vi "CPU_MEM_initialize_MEMs.vi"(8 "error in (no error)":errorcluster) -> (0 "error out":errorcluster)   [LabVIEW 2018]
uses:
  CPU_MEM_references.vi
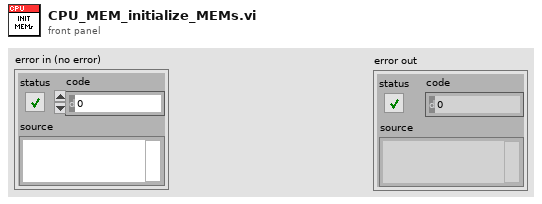
[diagram p1: front panel]
types:
  T1 = enum16{"init", "read DDR", "read PDR", "write DDR", "write PDR"}
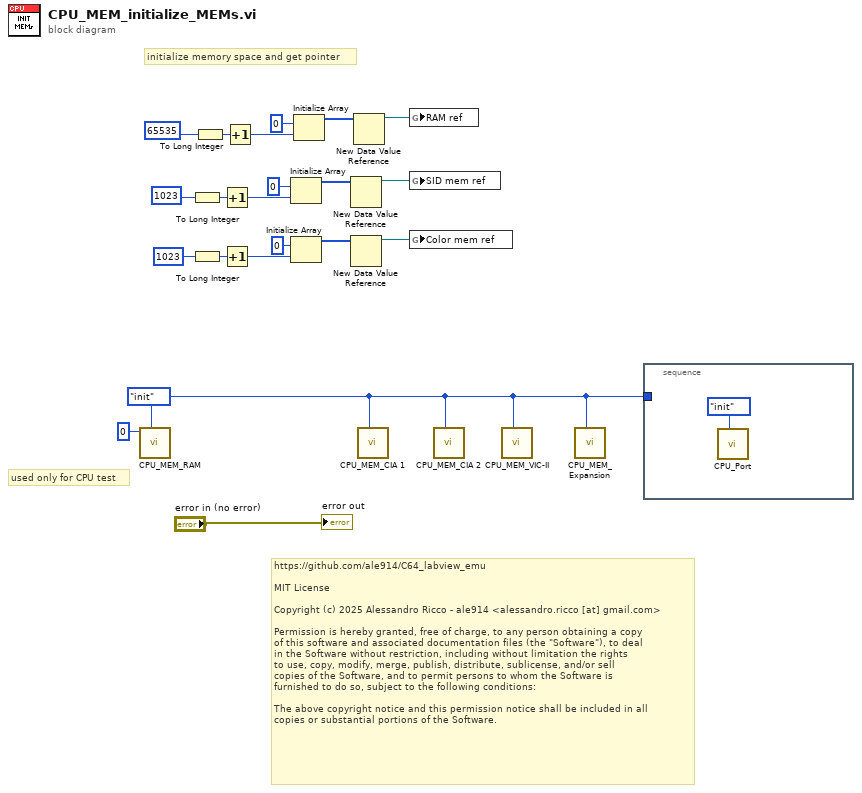
[diagram p0: block diagram]
diagram:
  w19 = enum16{"init", "read", "write"}."init" ("oper")
  # "used only for CPU test"
  # "initialize memory space and get pointer"
  # "https://github.com/ale914/C64_labview_emu\n\nMIT License\n\nCopyright (c) 2025 Alessandro Ricco - ale914 <alessandro.ricco [at] gmail.com>\n\nPermission is hereby granted, free of charge, to any person obtaining a copy\nof this software and associated documentation files (the \"Software\"), to deal\nin the Software without restriction, including without limitation the rights\nto use, copy, modify, merge, publish, distribute, sublicense, and/or sell\ncopies of the Software, and to permit persons to whom the Software is\nfurnished to do so, subject to the following conditions:\n\nThe above copyright notice and this permission notice shall be included in all\ncopies or substantial portions of the Software."
  n1 = call "CPU_MEM_RAM.vi"("oper"=w19, "address"=u16 0) -> ()  [unwired: 8 in, 2 out]
  n2 = To Long Integer(number=u16 1023 ("init size")) -> (32bit integer=w10:i32)
  n3 = To Long Integer(number=u16 1023 ("init size")) -> (32bit integer=w4:i32)
  n4 = To Long Integer(number=u16 65535 ("init size")) -> (32bit integer=w16:i32)
  n5 = Increment(x=w10) -> (x+1=w9:i32)
  n6 = Increment(x=w4) -> (x+1=w5:i32)
  n7 = Increment(x=w16) -> (x+1=w17:i32)
  n8 = Initialize Array(u8 0 ("element"), w9) -> (w11:u8[])
  n9 = Initialize Array(u8 0 ("element"), w5) -> (w3:u8[])
  n10 = Initialize Array(u8 0 ("element"), w17) -> (w15:u8[])
  n11 = New Data Value Reference(data value=w11) -> (data value reference=w12:refnum<data-value>)  [unwired: 1 in, 1 out]
  n12 = New Data Value Reference(data value=w3) -> (data value reference=w2:refnum<data-value>)  [unwired: 1 in, 1 out]
  n13 = New Data Value Reference(data value=w15) -> (data value reference=w14:refnum<data-value>)  [unwired: 1 in, 1 out]
  n14 = call "CPU_MEM_CIA 1.vi"("oper"=w19) -> ()  [unwired: 9 in, 2 out]
  n15 = global write "CPU_MEM_references.vi" "RAM ref"(w14) -> ()
  n16 = global write "CPU_MEM_references.vi" "SID mem ref"(w12) -> ()
  n17 = global write "CPU_MEM_references.vi" "Color mem ref"(w2) -> ()
  n18 = call "CPU_MEM_CIA 2.vi"("oper"=w19) -> ()  [unwired: 10 in, 1 out]
  n19 = call "CPU_MEM_VIC-II.vi"("oper"=w19) -> ()  [unwired: 9 in, 2 out]
  n20 = call "CPU_MEM_Expansion.vi"("oper"=w19) -> ()  [unwired: 10 in, 1 out]
  n21 = stacked-sequence {
    tunnel: w19 -> [_]
    frame #0 {
      n22 = call "CPU_Port.vi"("oper"=T1."init") -> ()  [unwired: 10 in, 1 out]
    }
  }
  "error out" <- "error in (no error)"
